vi "OrderPizza.vi"(8 "error in (no error)":errorcluster, 10 "PizzaId":T1, 11 "PizzaStore":refnum<class "PizzaStore.lvclass">) -> (0 "error out":errorcluster, 2 "Pizza":refnum<class "Pizza.lvclass">, 3 "PizzaStore":refnum<class "PizzaStore.lvclass">)   [LabVIEW 2020, in "FactoryMethod.lvlib" / "PizzaFactoryMethod.lvlib" / "PizzaStore.lvclass"]
uses:
  PizzaStore.lvclass
  TypeDef/PizzaId.ctl
  Pizza/Pizza.lvclass
  PizzaStore.lvclass/PizzaStore.ctl
  Support/Class/ConsoleOutput.lvclass
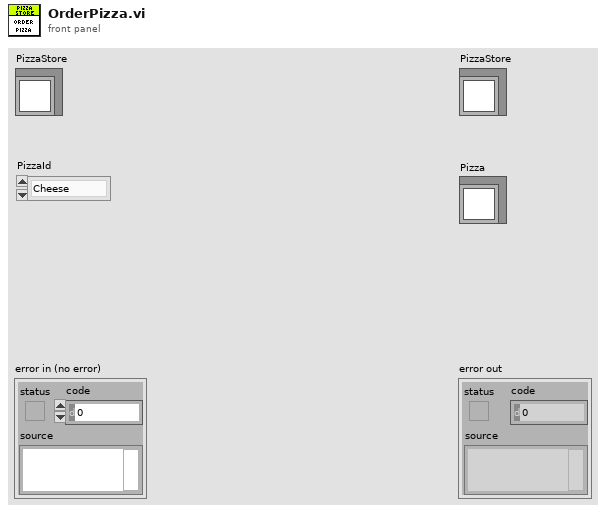
[diagram p1: front panel]
types:
  T1 = typedef "FactoryMethod.lvlib/PizzaFactoryMethod.lvlib/PizzaStore.lvclass/PizzaId.ctl" = enum16{"Cheese", "Clam", "Pepperoni", "Veggie"}
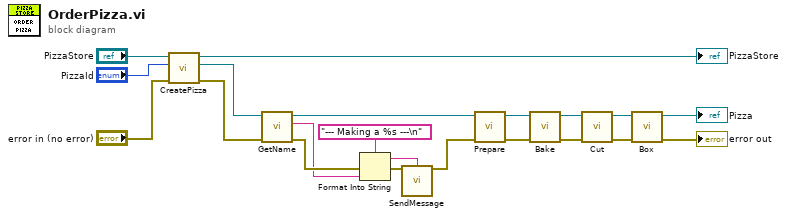
[diagram p0: block diagram]
diagram:
  n1 = call-dynamic "CreatePizza.vi"("error in (no error)"="error in (no error)", "PizzaId"="PizzaId", "PizzaStore"="PizzaStore") -> ("error out"=w7:errorcluster, "Pizza"=w8:refnum<class "Pizza.lvclass">, "PizzaStore"=→"PizzaStore":refnum<class "PizzaStore.lvclass">)  [unwired: 6 in]
  n2 = call "GetName.vi"("error in (no error)"=w7, "Pizza in"=w8) -> ("error out"=w5:errorcluster, "Name"=w4:string, "Pizza out"=w6:refnum<class "Pizza.lvclass">)  [unwired: 7 in]
  n3 = Format Into String(format string="--- Making a %s ---\n", error in=w5, w4) -> (resulting string=w1:string, error out=w2:errorcluster)  [unwired: 1 in]
  n4 = call "SendMessage.vi"("Message"=w1, "error in (no error)"=w2) -> ("error out"=w9:errorcluster)  [unwired: 13 in]
  n5 = call "Prepare.vi"("error in (no error)"=w9, "Pizza in"=w6) -> ("error out"=w12:errorcluster, "Pizza out"=w13:refnum<class "Pizza.lvclass">)  [unwired: 8 in]
  n6 = call-dynamic "Bake.vi"("error in (no error)"=w12, "Pizza in"=w13) -> ("error out"=w15:errorcluster, "Pizza out"=w14:refnum<class "Pizza.lvclass">)  [unwired: 8 in]
  n7 = call-dynamic "Cut.vi"("error in (no error)"=w15, "Pizza in"=w14) -> ("error out"=w17:errorcluster, "Pizza out"=w16:refnum<class "Pizza.lvclass">)  [unwired: 8 in]
  n8 = call "Box.vi"("error in (no error)"=w17, "Pizza in"=w16) -> ("error out"=→"error out":errorcluster, "Pizza out"=→"Pizza":refnum<class "Pizza.lvclass">)  [unwired: 8 in]
